vi "optotrak.vi"(10 "Position Convention":u16, 11 "Data File in":T1) -> (1 "mse":dbl format="%.2f", 2 "Coefficients":dbl[][](array[numeric]) format="%.2f", 3 "Data File out":T1)   [LabVIEW 2016]
uses:
  <vilib>/Analysis/baseanly.llb/Real A x B.vi
  <vilib>/Analysis/baseanly.llb/Real Inverse Matrix.vi
  comm/quaternion/quaternion.lvlib
  comm/fick-matrix/fick-matrix.lvlib
  <vilib>/Analysis/NI_AALBase.lvlib
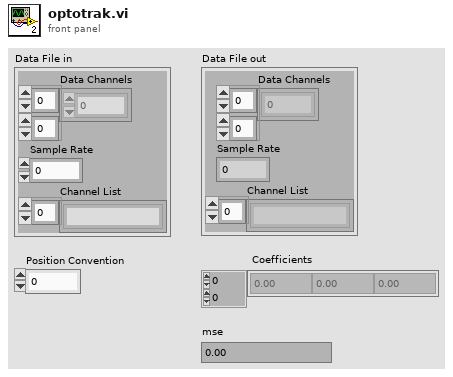
[diagram p1: front panel]
types:
  T1 = cluster{"Data Channels":dbl[][], "Sample Rate":i32, "Channel List":string[]}
  T2 = typedef "NI_Matrix.lvlib/RealMatrix.ctl" = dbl[][]
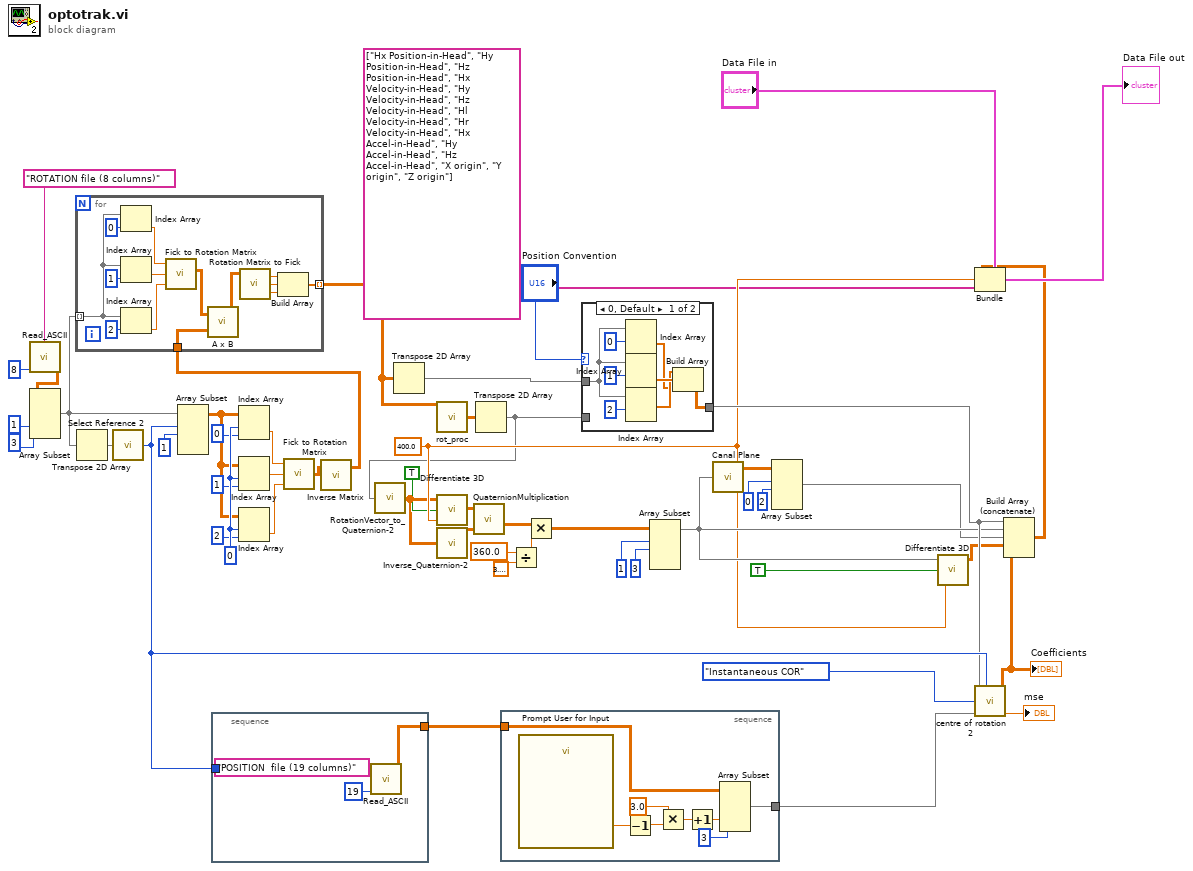
[diagram p0: block diagram]
diagram:
  w36 = 0 ("disabled index (col)")
  w20 = 400.0 ("Sample Rate")
  n1 = call "Read_ASCII.vi"("Number of Columns"=8, "Prompt"="ROTATION file (8 columns)") -> ("Output"=w46:sgl[][])  [unwired: 7 in]
  n2 = Array Subset(array=w46, index (col)=1 ("index"), length (col)=3 ("length")) -> (w29:sgl[][])  [unwired: 2 in]
  n3 = Transpose 2D Array(2D array=w29) -> (transposed array=w32:sgl[][])
  n4 = call "Select Reference 2.vi"("3D Coil"=w32) -> ("Element Data"=w51:i32)
  n5 = Array Subset(array=w29, index (row)=w51, length (row)=1 ("length")) -> (w25:sgl[][])  [unwired: 2 in]
  n6 = stacked-sequence {
    tunnel: [w54] -> w50
    tunnel: w51 -> [_]
    frame #0 {
      n7 = call "Read_ASCII.vi"("Number of Columns"=19, "Prompt"="POSITION  file (19 columns)") -> ("Output"=w54:sgl[][])  [unwired: 7 in]
    }
  }
  n8 = Index Array(array=w25, index (row)=w36, index (col)=0 ("index (row)")) -> (element=w26:sgl)
  n9 = Index Array(array=w25, index (row)=w36, index (col)=1 ("index (row)")) -> (element=w27:sgl)
  n10 = Index Array(array=w25, index (row)=w36, index (col)=2 ("index (row)")) -> (element=w28:sgl)
  n11 = call "Fick to Rotation Matrix.vi"("T"=w28, "V"=w27, "H"=w26) -> ("Rotation Matrix"=w30:dbl[][])
  n12 = call-poly <vilib>:"Inverse Matrix.vi"("Input Matrix"=w30) -> ("Inverse Matrix"=w31:T2)  [unwired: 1 in, 1 out]
  n13 = for {
    tunnel: w29 -> [w64] mode=indexing
    tunnel: w31 -> [w63]
    tunnel: [w57] -> w38 mode=indexing
    n14 = Index Array(array=w64, index=0 ("index (row)")) -> (element=w68:sgl)
    n15 = Index Array(array=w64, index=1 ("index (row)")) -> (element=w69:sgl)
    n16 = Index Array(array=w64, index=2 ("index (row)")) -> (element=w70:sgl)
    n17 = call "Fick to Rotation Matrix.vi"("T"=w70, "V"=w69, "H"=w68) -> ("Rotation Matrix"=w62:dbl[][])
    n18 = call-poly <vilib>:"A x B.vi"("B"=w63, "A"=w62) -> ("A x B"=w61:T2)  [unwired: 1 out]
    n19 = call "Rotation Matrix to Fick.vi"("A"=w61) -> ("T"=w58:dbl, "V"=w59:dbl, "H"=w60:dbl)  [unwired: 2 in]
    n20 = Build Array(w60, w59, w58) -> (w57:dbl[])
  }
  n21 = Transpose 2D Array(2D array=w38) -> (transposed array=w37:dbl[][])
  n22 = call "rot_proc.vi"("Euler Angles"=w38) -> ("Rotation Vectors"=w17:dbl[][])  [unwired: 17 in, 1 out]
  n23 = Transpose 2D Array(2D array=w17) -> (transposed array=w18:dbl[][])
  n24 = call "RotationVector_to_Quaternion-2.vi"("rotation vectors"=w18) -> ("quaternions"=w12:dbl[][])  [unwired: 4 in]
  n25 = call "Differentiate 3D.vi"("Sample Rate 4"=w20, "Fixed Sample Rate"=TRUE, "Data (in)"=w12) -> ("Data (differentiated)"=w3:dbl[][])  [unwired: 2 in]
  n26 = call "Inverse_Quaternion-2.vi"("quaternions"=w12) -> ("inverse quaternions"=w4:dbl[][])  [unwired: 4 in]
  n27 = call "QuaternionMultiplication.vi"("quaternions B"=w4, "quaternions A"=w3) -> ("quaternions A x B"=w5:dbl[][])  [unwired: 3 in]
  n28 = stacked-sequence {
    tunnel: [w72] -> w49
    tunnel: w50 -> [w71]
    frame #0 {
      n29 = call "Prompt User for Input"() -> ("LED"=w77:dbl)  [unwired: 17 in, 2 out]
      n30 = Decrement(x=w77) -> (x-1=w76:dbl)
      n31 = Multiply(x=3.0, y=w76) -> (x*y=w74:dbl)
      n32 = Increment(x=w74) -> (x+1=w73:dbl)
      n33 = Array Subset(array=w71, index (col)=w73, length (col)=3 ("length")) -> (w72:sgl[][])  [unwired: 2 in]
    }
  }
  n34 = Divide(x=360.0, y=3.141592653589793) -> (x/y=w8:dbl)
  n35 = Multiply(x=w5, y=w8) -> (x*y=w41:dbl[][])
  n36 = case shown="0, Default" "Position Convention" {
    tunnel: w37 -> [w86 _]
    tunnel: w18 -> [_ w87]
    tunnel: [w79 w87] -> w44
    frame 0, Default {
      n37 = Index Array(array=w86, index (row)=0) -> (element=w80:dbl[])  [unwired: 1 in]
      n38 = Index Array(array=w86, index (row)=1) -> (element=w82:dbl[])  [unwired: 1 in]
      n39 = Index Array(array=w86, index (row)=2) -> (element=w81:dbl[])  [unwired: 1 in]
      n40 = Build Array(w81, w82, w80) -> (w79:dbl[][])
    }
    frame 1 {
    }
  }
  n41 = Array Subset(array=w41, index (row)=1 ("Array Index"), length (row)=3 ("Array Index")) -> (w42:dbl[][])  [unwired: 2 in]
  n42 = call "Canal Plane.vi"("Principal Planes"=w42) -> ("Canal Planes"=w9:dbl[][])
  n43 = Array Subset(array=w9, index (row)=0 ("Array Index"), length (row)=2 ("Array Index")) -> (w15:dbl[][])  [unwired: 2 in]
  n44 = call "Differentiate 3D.vi"("Sample Rate 4"=w20, "Fixed Sample Rate"=TRUE, "Data (in)"=w42) -> ("Data (differentiated)"=w16:dbl[][])  [unwired: 2 in]
  n45 = call "centre of rotation 2.vi"("Head rotation (Fick)"=w44, "reference"=w51, "Analysis"=enum16{"Instantaneous COR", "Average COR"}."Instantaneous COR", "POSITION 3D"=w49) -> ("Coefficients"=w45:dbl[][], "mse"=→"mse":dbl)  [unwired: 10 in]
  "Coefficients" <- w45
  n46 = Build Array (concatenate)(w44, w42, w15, w16, w45) -> (w19:dbl[][])
  n47 = Bundle(cluster="Data File in", "Data Channels"=w19, "Sample Rate"=w20, "Channel List"=string[] ["Hx Position-in-Head", "Hy Position-in-Head", "Hz Position-in-Head", "Hx Velocity-in-Head", "Hy Velocity-in-Head", "Hz Velocity-in-Head", "Hl Velocity-in-Head", "Hr Velocity-in-Head", "Hx Accel-in-Head", "Hy Accel-in-Head", "Hz Accel-in-Head", "X origin", "Y origin", "Z origin"]) -> (→"Data File out":T1)
